vi "FrameToPose.vi"(1 "Frame":T2 {"Pw" format="%.2f"; "Pz" format="%.2f"; "Py" format="%.2f"; "Px" format="%.2f"; "aw" format="%.2f"; "az" format="%.2f"; "ay" format="%.2f"; "ax" format="%.2f"; "ow" format="%.2f"; "nw" format="%.2f"; "oz" format="%.2f"; "oy" format="%.2f"; "ox" format="%.2f"; "nz" format="%.2f"; "ny" format="%.2f"; "nx" format="%.2f"}) -> (0 "Pose":T1)   [LabVIEW 2012]
uses:
  <userlib>/rosforlv/Gazebo/AxesDrawing/ReferenceFrame.ctl
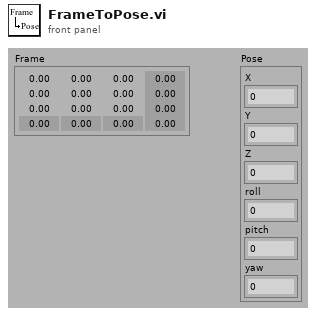
[diagram p1: front panel]
types:
  T1 = cluster{"X":sgl, "Y":sgl, "Z":sgl, "roll":sgl, "pitch":sgl, "yaw":sgl}
  T2 = typedef "ReferenceFrame.ctl" = cluster{"nx":dbl, "ny":dbl, "nz":dbl, "nw":dbl, "ox":dbl, "oy":dbl, "oz":dbl, "ow":dbl, "ax":dbl, "ay":dbl, "az":dbl, "aw":dbl, "Px":dbl, "Py":dbl, "Pz":dbl, "Pw":dbl}
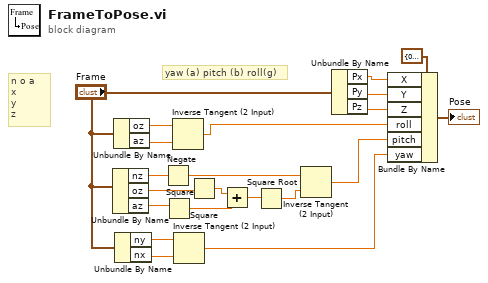
[diagram p0: block diagram]
diagram:
  # "yaw (a) pitch (b) roll(g)"
  # "n o a\nx\ny\nz"
  n1 = Unbundle By Name("Frame") -> ("nz"=w8:dbl, "oz"=w11:dbl, "az"=w10:dbl)
  n2 = Unbundle By Name("Frame") -> ("oz"=w17:dbl, "az"=w16:dbl)
  n3 = Unbundle By Name("Frame") -> ("ny"=w6:dbl, "nx"=w7:dbl)
  n4 = Negate(x=w8) -> (-x=w9:dbl)
  n5 = Square(x=w10) -> (x^2=w13:dbl)
  n6 = Inverse Tangent (2 Input)(1:w16, 2:w17) -> (0:w18:dbl)
  n7 = Inverse Tangent (2 Input)(1:w7, 2:w6) -> (0:w20:dbl)
  n8 = Square(x=w11) -> (x^2=w12:dbl)
  n9 = Add(x=w12, y=w13) -> (x+y=w14:dbl)
  n10 = Square Root(x=w14) -> (sqrt(x)=w15:dbl)
  n11 = Inverse Tangent (2 Input)(1:w15, 2:w9) -> (0:w19:dbl)
  n12 = Unbundle By Name("Frame") -> ("Px"=w3:dbl, "Py"=w4:dbl, "Pz"=w5:dbl)
  n13 = Bundle By Name(cluster=T1 {"X"=0.0, "Y"=0.0, "Z"=0.0, "roll"=0.0, "pitch"=0.0, "yaw"=0.0} ("Pose"), "X"=w3, "Y"=w4, "Z"=w5, "roll"=w18, "pitch"=w19, "yaw"=w20) -> (→"Pose":T1)
